vi "Marker.vi"(9 "Markers in":string[][](array[string]), 10 "Initial String":string) -> (1 "Markers out":string[][](array[string]), 3 "Balloon":string)   [LabVIEW 2012]
doc: "This VI creates a marker URL format"
panel:
  in  "Character":string(combo)
  in  "Cancel":bool
  in  "Add Marker":bool
  out "Add Another?":bool
  in  "Color":string(combo)
  in  "Size":string(combo)
  in  "Longitude":dbl format="%#.6g"
  in  "Latitude":dbl format="%#.6g"
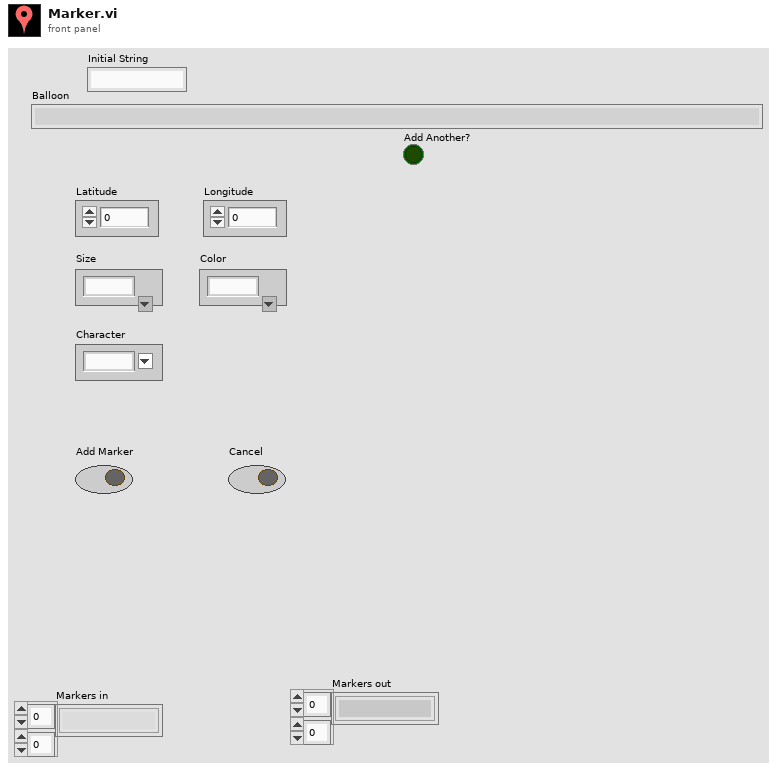
[diagram p1: front panel]
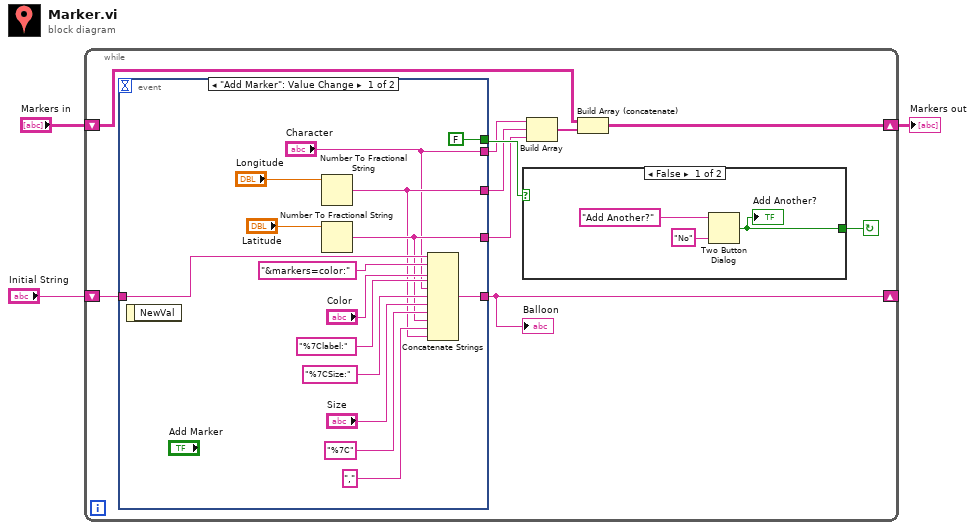
[diagram p0: block diagram]
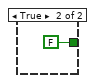
[diagram p2: hidden frame]
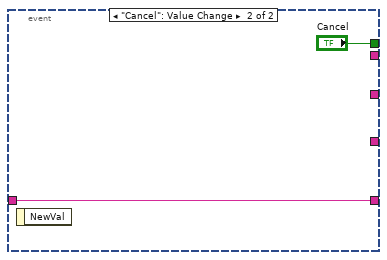
[diagram p3: hidden frame]
diagram:
  n1 = while {
    shift-right: [w10] -> _
    shift-left: "Initial String" -> [w13]
    shift-right: [w5] -> w2
    shift-left: "Markers in" -> [w4]
    stop <- w12 continue-if-true
    n2 = event shown="[0] \"Add Marker\": Value Change" {
      selector: _ -> [_ _]
      dyn-events: _ -> [_ _]
      timeout: _ -> [_ _]
      tunnel: [w26 w34] -> w10
      tunnel: w13 -> [w25 w34]
      tunnel: [FALSE ("Cancel") "Cancel"] -> w11
      tunnel: [w20 _] -> w7
      tunnel: [w19 _] -> w8
      tunnel: ["Character" _] -> w9
      event "Add Marker": Value Change {
        n3 = event-data() -> ()  [unwired: 1 in, 1 out]
        n4 = Number To Fractional String(number="Longitude") -> (F-format string=w19:string)  [unwired: 3 in]
        n5 = Number To Fractional String(number="Latitude") -> (F-format string=w20:string)  [unwired: 3 in]
        n6 = Concatenate Strings(w25, "&markers=color:", "Color", "%7Clabel:" ("string"), "Character", "%7CSize:" ("string"), "Size", "%7C" ("string"), w20, ",", w19) -> (w26:string)
      }
      event "Cancel": Value Change {
        n7 = event-data() -> ()  [unwired: 1 in, 1 out]
      }
    }
    "Balloon" <- w10
    n8 = case shown="False" w11 {
      tunnel: [w16 FALSE ("T button?")] -> w12
      frame False {
        n9 = Two Button Dialog(message="Add Another?", 1:"No" ("F button name (\"Cancel\")")) -> (T button?=w16:bool)  [unwired: 1 in]
        "Add Another?" <- w16
      }
      frame True {
      }
    }
    n10 = Build Array(w9, w8, w7) -> (w6:string[])
    n11 = Build Array (concatenate)(w4, w6) -> (w5:string[][])
  }
  "Markers out" <- w2
